vi "Get User Interface VI.vi"(8 "error in (no error)":errorcluster, 11 "Core Group User Interface in":refnum<class "Core Group User Interface.lvclass">) -> (0 "error out":errorcluster, 2 "user interface vi":refnum<vi>, 3 "Core Group User Interface out":refnum<class "Core Group User Interface.lvclass">)   [LabVIEW 2019, in "DSF Core.lvlib" / "Core Group User Interface.lvclass"]
uses:
  Core Group User Interface.lvclass
  User Interface.vi
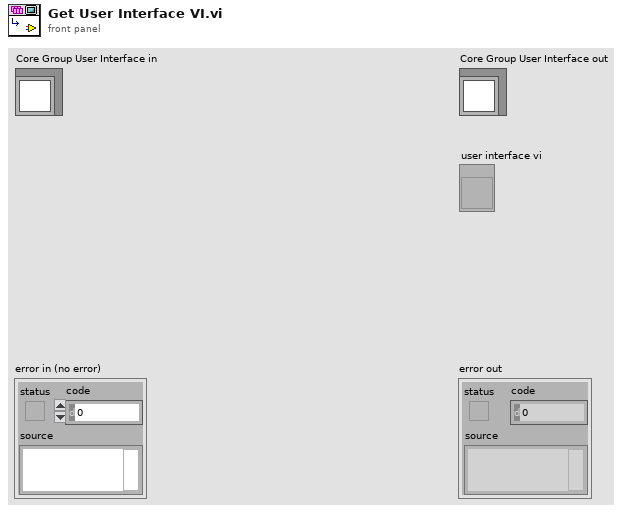
[diagram p1: front panel]
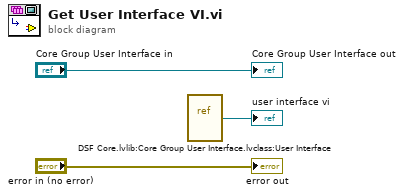
[diagram p0: block diagram]
diagram:
  n1 = vi-ref "DSF Core.lvlib:Core Group User Interface.lvclass:User Interface.vi"() -> (→"user interface vi":refnum<vi>)
  "error out" <- "error in (no error)"
  "Core Group User Interface out" <- "Core Group User Interface in"
